vi "Get Instrument Identifier.vi"(11 "CFG Base in":refnum<class "CFG Base.lvclass">) -> (2 "Instrument Identifier":string, 3 "CFG Base out":refnum<class "CFG Base.lvclass">)   [LabVIEW 2024, in "HAL.lvlib" / "CFG Base.lvclass"]
uses:
  CFG Base.lvclass
  CFG Base.lvclass/CFG Base.ctl
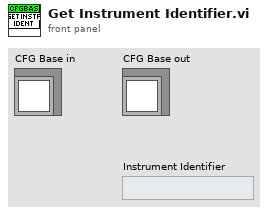
[diagram p1: front panel]
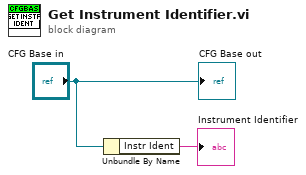
[diagram p0: block diagram]
diagram:
  n1 = Unbundle By Name("CFG Base in") -> ("Instr Ident"=→"Instrument Identifier":string)
  "CFG Base out" <- "CFG Base in"
